vi "MethodTest.vi"() -> ()   [LabVIEW 2018, in "HttpExamples.lvlib"]
uses:
  Types/method_enum.ctl
  HttpHeaders_response/HttpHeaders_Response.lvclass
  C:/Viviota/Projects/R&D/LabVIEW_HTTP_REST_NET/HTTPHeaders_NET/HttpHeaders_NET.lvclass
  HttpHeaders_content/HttpHeaders_Content.lvclass
  HTTPHeaders_NET/HttpHeaders_NET.lvclass
  HttpExamples.lvlib
  LabVIEWHTTPClient_NET/LabVIEWHTTPClient_NET.lvclass
  LabVIEWHTTPClient_NET.lvlib
panel:
  out "ReasonPhrase":string
  out "StatusCode":i32(ring)=100 items=["Continue"=100, "SwitchingProtocols"=101, "OK"=200, "Created"=201, "Accepted"=202, "NonAuthoritativeInformation"=203, "NoContent"=204, "ResetContent"=205, "PartialContent"=206, "MultipleChoices, Ambiguous"=300, "MovedPermanently, Moved"=301, "Found, Redirect"=302, "SeeOther, RedirectMethod"=303, "NotModified"=304, "UseProxy"=305, "Unused"=306, "TemporaryRedirect, RedirectKeepVerb"=307, "BadRequest"=400, "Unauthorized"=401, "PaymentRequired"=402, "Forbidden"=403, "NotFound"=404, "MethodNotAllowed"=405, "NotAcceptable"=406, "ProxyAuthenticationRequired"=407, "RequestTimeout"=408, "Conflict"=409, "Gone"=410, "LengthRequired"=411, "PreconditionFailed"=412, "RequestEntityTooLarge"=413, "RequestUriTooLong"=414, "UnsupportedMediaType"=415, "RequestedRangeNotSatisfiable"=416, "ExpectationFailed"=417, "UpgradeRequired"=426, "InternalServerError"=500, "NotImplemented"=501, "BadGateway"=502, "ServiceUnavailable"=503, "GatewayTimeout"=504, "HttpVersionNotSupported"=505]
  in  "Method":T1
  out "Header Values":string[](array[string])
  out "Header Names":string[](array[string])
  in  "request headers":cluster{"header":string, "value":string}[](array[cluster])
  out "error out":errorcluster
  out "Response":string
  in  "buffer":string
  in  "URL":string
  # "http://httpbin.org"
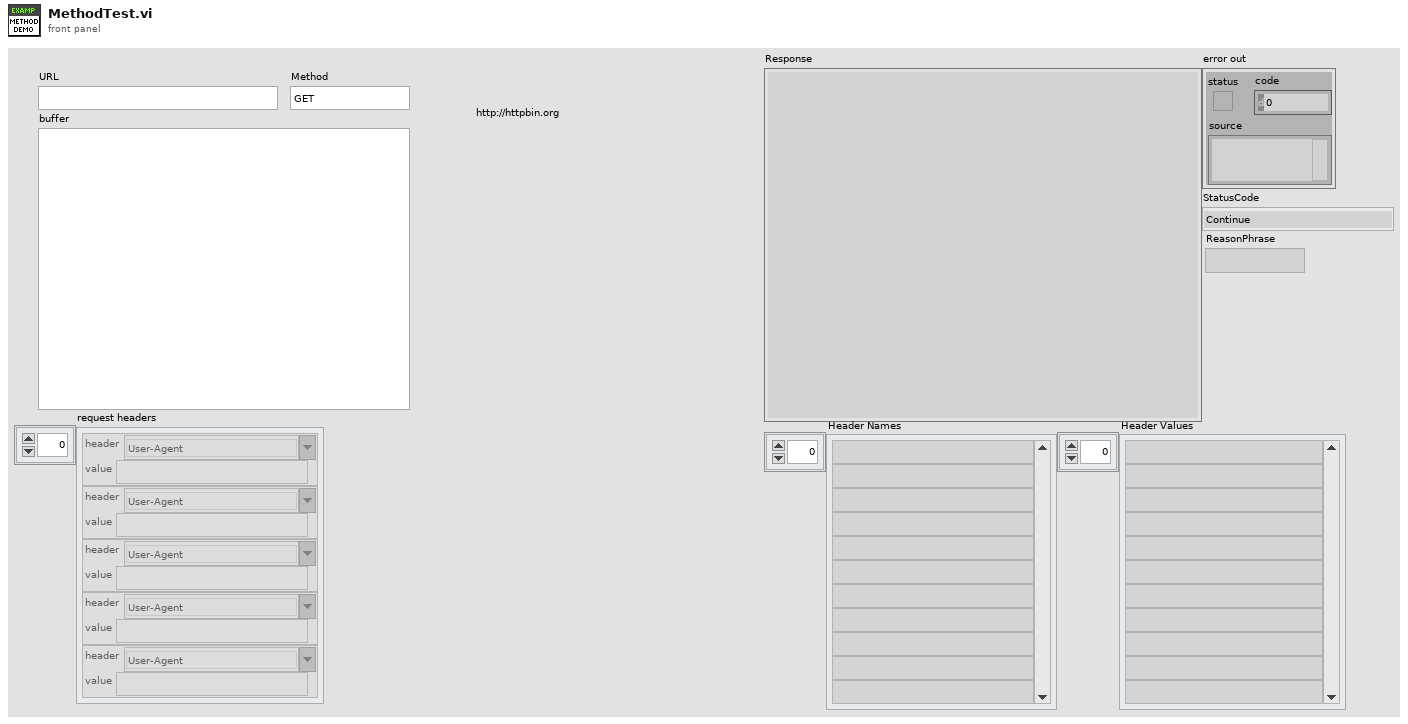
[diagram p1: front panel]
types:
  T1 = typedef "LabVIEWHTTPClient_NET.lvlib/method_enum.ctl" = enum16{"GET", "PUT", "POST", "DELETE", "HEAD", "TRACE", "SEND"}
  T2 = typedef "LabVIEWHTTPClient_NET.lvlib/ResponseHeaders_Cluster.ctl" = cluster{"ResponseHeader":refnum<class "HttpHeaders_Response.lvclass">, "ContentHeaders":refnum<class "HttpHeaders_Content.lvclass">}
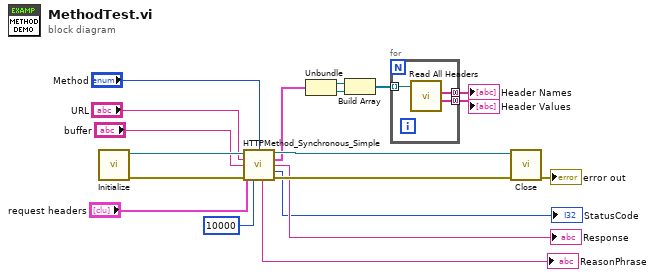
[diagram p0: block diagram]
diagram:
  n1 = call "Initialize.vi"() -> ("error out"=w17:errorcluster, "HTTP Client Out"=w19:refnum<class "LabVIEWHTTPClient_NET.lvclass">)  [unwired: 10 in]
  n2 = call "HTTPMethod_Synchronous_Simple.vi"("LabVIEWHTTPClient_NET in"=w19, "Method"="Method", "URL"="URL", "buffer"="buffer", "request headers"="request headers", "error in (no error)"=w17, "Timeout_ms (10000)"=10000) -> ("LabVIEWHTTPClient_NET out"=w18:refnum<class "LabVIEWHTTPClient_NET.lvclass">, "Headers"=w8:T2, "Response"=→"Response":string, "StatusCode"=→"StatusCode":i32, "ReasonPhrase"=→"ReasonPhrase":string, "error out"=w16:errorcluster)  [unwired: 2 in, 1 out]
  n3 = Unbundle(w8) -> ("ResponseHeader"=w6:refnum<class "HttpHeaders_Response.lvclass">, "ContentHeaders"=w7:refnum<class "HttpHeaders_Content.lvclass">)
  n4 = Build Array(w6, w7) -> (w5:refnum<class "HttpHeaders_NET.lvclass">[])
  n5 = for {
    tunnel: w5 -> [w22] mode=indexing
    tunnel: [w21] -> w4 mode=concatenating
    tunnel: [w20] -> w3 mode=concatenating
    n6 = call-dynamic "Read All Headers.vi"("HTTPHeaders_NET in"=w22) -> ("Header Values"=w20:string[], "Header Names"=w21:string[])  [unwired: 7 in, 2 out]
  }
  "Header Names" <- w4
  "Header Values" <- w3
  n7 = call "Close.vi"("Error In"=w16, "LabVIEWHTTPClient_NET in"=w18) -> ("Error Out"=→"error out":errorcluster)  [unwired: 9 in]
